vi "Single Button Pressed.vi"(11 "Button Value":bool) -> (3 "Button Press":bool)   [LabVIEW 2017]
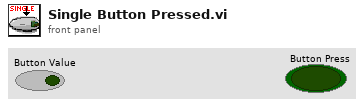
[diagram p1: front panel]
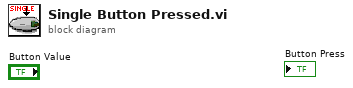
[diagram p0: block diagram]
diagram:
